vi "SEK2020v1VI1IrAteFinalDoCampo.vi"(8 "Parâmetros":T1={"Azul Max EV3 Cor"=17, "Azul Min EV3 Cor"=0, "Verde Max EV3 Cor"=6.0, "Verde Min EV3 Cor"=0.0, "Vermelho Max Ev3 Cor"=0, "Vermelho Min EV3 Cor"=0, "Chão EV3 Cor"=0.0, "Branco Max EV3 Cor"=0.0, "Branco Min EV3 Cor"=0.0, "Preto Max EV3 Cor"=0.0, "Preto Min EV3 Cor"=0.0, "Distância Tubulação"=0.0, "Distância Frontal"=0.0, "Amarelo Max EV3 Cor"=0.0, "Amarelo Min EV3 Cor"=0.0, "Distância Lateral"=0.0, "90°"=0.0, "180°"=0.0, "Seguidor de Linha"=0.0}, 10 "NXT/EV3":T2) -> (2 "NXT/EV3 2":T2)   [LabVIEW 2016]
uses:
  <vilib>/NXT/Subs/LVHSConnector.ctl
  <vilib>/NXT/LegoClasses/BrickReference/BrickReference.lvclass
  <vilib>/NXT/Block Support/NXT_OutputPort.ctl
  <vilib>/NXT/Block Support/NXT_InputPort.ctl
  <vilib>/NXT/Dual Mode Library/Sensors/EV3_Color_Reflect.vi
  <vilib>/NXT/NXTIO Xnodes/NXTIONodeSubVIs/NXTStopMotors.vi
  <vilib>/NXT/NXTIO Xnodes/AddressXNode/NXTIOAddress.xnode
  <vilib>/NXT/NXTIO Xnodes/NXTIOXNode/NXTIO.xnode
panel:
  # "Sensor EV3 Cor"
  # "Sensor Ultrassônico"
  # "Sensor Giroscópio"
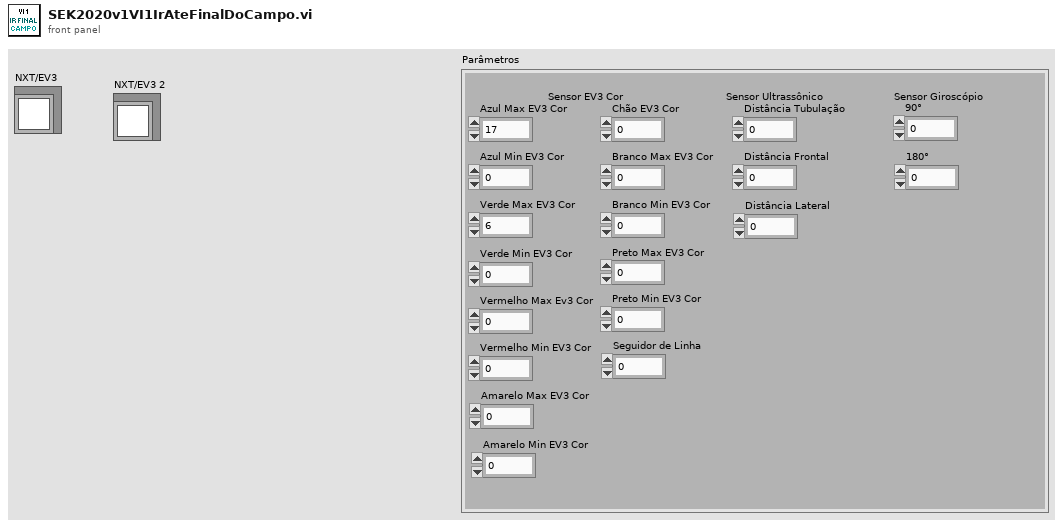
[diagram p1: front panel]
types:
  T1 = cluster{"Azul Max EV3 Cor":i32, "Azul Min EV3 Cor":i32, "Verde Max EV3 Cor":dbl, "Verde Min EV3 Cor":dbl, "Vermelho Max Ev3 Cor":i32, "Vermelho Min EV3 Cor":i32, "Chão EV3 Cor":sgl, "Branco Max EV3 Cor":sgl, "Branco Min EV3 Cor":sgl, "Preto Max EV3 Cor":sgl, "Preto Min EV3 Cor":sgl, "Distância Tubulação":sgl, "Distância Frontal":sgl, "Amarelo Max EV3 Cor":dbl, "Amarelo Min EV3 Cor":dbl, "Distância Lateral":sgl, "90°":sgl, "180°":sgl, "Seguidor de Linha":dbl}
  T2 = typedef "LVHSConnector.ctl" = refnum<class "BrickReference.lvclass">
  T3 = typedef "NXT_InputPort.ctl" = u32
  T4 = typedef "NXT_OutputPort.ctl" = u8
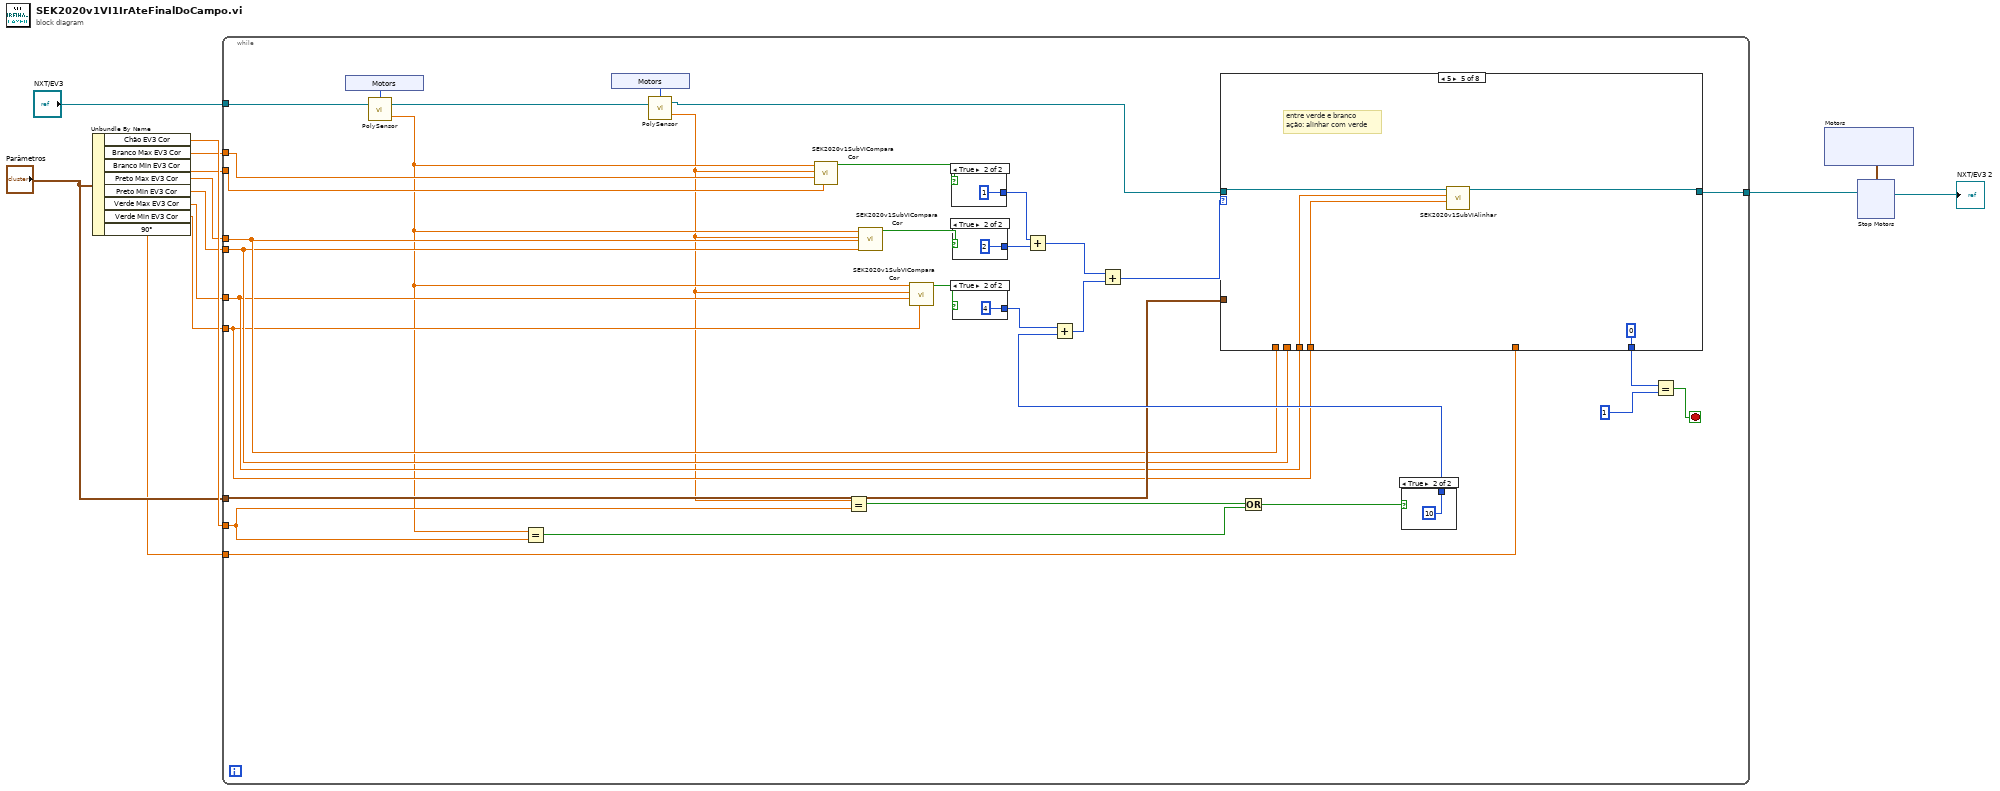
[diagram p0: block diagram]
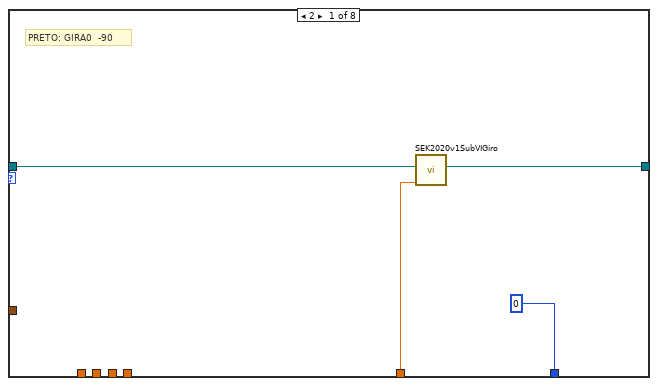
[diagram p2: hidden frame]
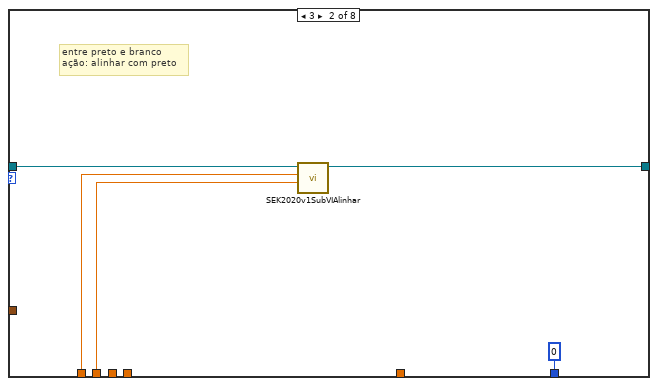
[diagram p3: hidden frame]
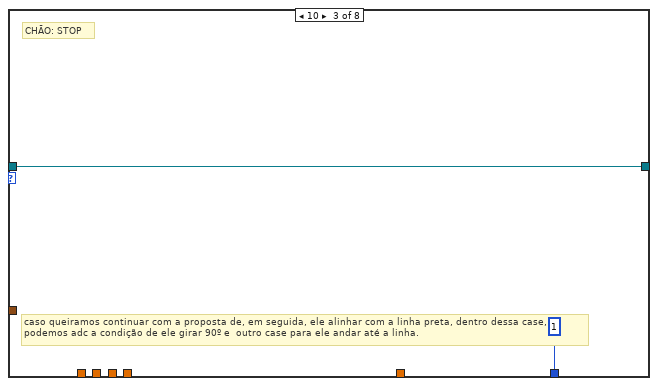
[diagram p4: hidden frame]
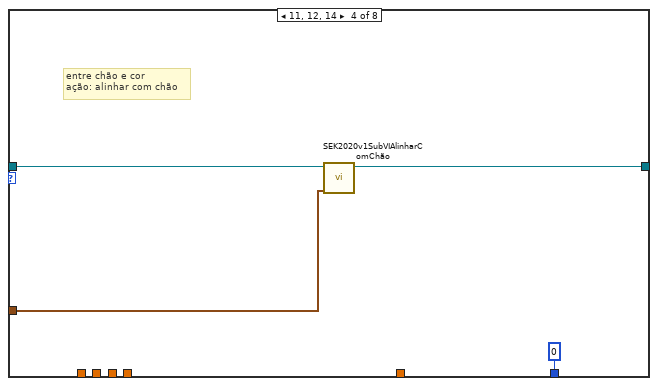
[diagram p5: hidden frame]
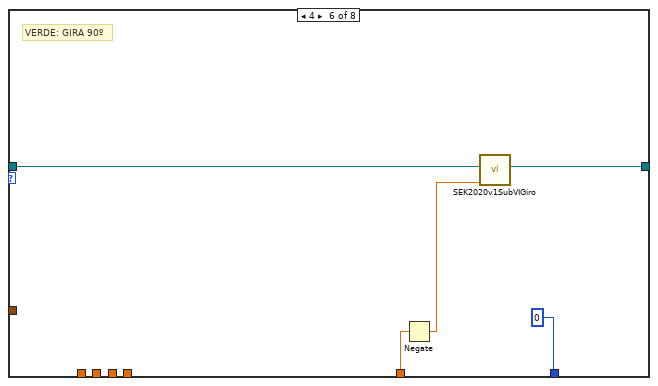
[diagram p6: hidden frame]
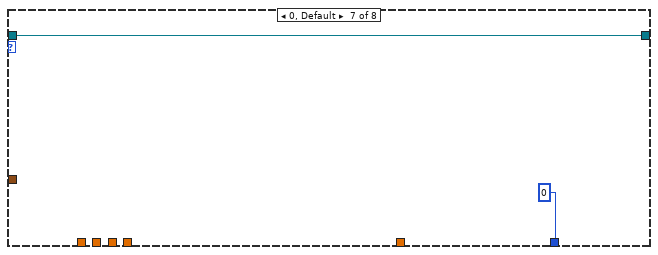
[diagram p7: hidden frame]
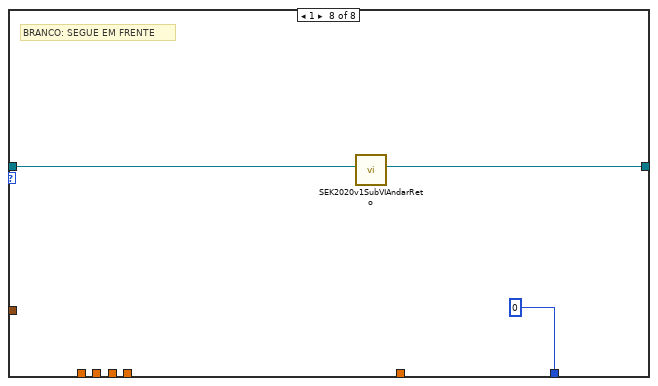
[diagram p8: hidden frame]
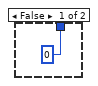
[diagram p9: hidden frame]
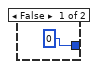
[diagram p10: hidden frame]
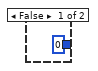
[diagram p11: hidden frame]
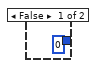
[diagram p12: hidden frame]
diagram:
  n1 = Unbundle By Name("Parâmetros") -> ("Chão EV3 Cor"=w12:sgl, "Branco Max EV3 Cor"=w5:sgl, "Branco Min EV3 Cor"=w8:sgl, "Preto Max EV3 Cor"=w4:sgl, "Preto Min EV3 Cor"=w7:sgl, "Verde Max EV3 Cor"=w3:dbl, "Verde Min EV3 Cor"=w6:dbl, "90°"=w1:sgl)
  n2 = while {
    tunnel: "NXT/EV3" -> [w34]
    tunnel: w12 -> [w21]
    tunnel: [w37] -> w9
    tunnel: w8 -> [w24]
    tunnel: w7 -> [w22]
    tunnel: w6 -> [w18]
    tunnel: w5 -> [w25]
    tunnel: w4 -> [w23]
    tunnel: w3 -> [w19]
    tunnel: "Parâmetros" -> [w26]
    tunnel: w1 -> [w14]
    stop <- w33 stop-if-true
    n3 = xnode "Motors"() -> ("Sensor"=w45:T3)
    n4 = call-poly <vilib>:"PolySensor.vi"("NXT/EV3"=w34, "Port (Port 1)"=w45) -> ("Scaled Value"=w17:sgl, "NXT/EV3"=w35:T2)  [unwired: 1 in]
    n5 = Equal?(x=w17, y=w21) -> (x = y?=w32:bool)
    n6 = xnode "Motors"() -> ("Sensor"=w46:T3)
    n7 = call-poly <vilib>:"PolySensor.vi"("NXT/EV3"=w35, "Port (Port 1)"=w46) -> ("Scaled Value"=w16:sgl, "NXT/EV3"=w15:T2)  [unwired: 1 in]
    n8 = call "SEK2020v1SubVIComparaCor.vi"("Branco Min EV3 Cor"=w24, "Branco Max EV3 Cor"=w25, "Scaled Value 2"=w16, "Scaled Value"=w17) -> ("Boolean"=w29:bool)  [unwired: 7 in]
    n9 = Equal?(x=w16, y=w21) -> (x = y?=w44:bool)
    n10 = call "SEK2020v1SubVIComparaCor.vi"("Branco Min EV3 Cor"=w22, "Branco Max EV3 Cor"=w23, "Scaled Value 2"=w16, "Scaled Value"=w17) -> ("Boolean"=w28:bool)  [unwired: 7 in]
    n11 = call "SEK2020v1SubVIComparaCor.vi"("Branco Min EV3 Cor"=w18, "Branco Max EV3 Cor"=w19, "Scaled Value 2"=w16, "Scaled Value"=w17) -> ("Boolean"=w27:bool)  [unwired: 7 in]
    n12 = case shown="True" w29 {
      tunnel: [0 1] -> w43
      frame False {
      }
      frame True {
      }
    }
    n13 = case shown="True" w28 {
      tunnel: [0 2] -> w42
      frame False {
      }
      frame True {
      }
    }
    n14 = case shown="True" w27 {
      tunnel: [0 4] -> w38
      frame False {
      }
      frame True {
      }
    }
    n15 = Add(x=w43, y=w42) -> (x+y=w39:i32)
    n16 = Or(x=w44, y=w32) -> (x .or. y?=w36:bool)
    n17 = case shown="True" w36 {
      tunnel: [0 10] -> w41
      frame False {
      }
      frame True {
      }
    }
    n18 = Add(x=w38, y=w41) -> (x+y=w40:i32)
    n19 = Add(x=w39, y=w40) -> (x+y=w20:i32)
    n20 = case shown="5" w20 {
      tunnel: [w49 w53 w56 w61 w66 w70 w72 w75] -> w37
      tunnel: [0 0 1 0 0 0 0 0] -> w30
      tunnel: w23 -> [_ w55 _ _ _ _ _ _]
      tunnel: w22 -> [_ w54 _ _ _ _ _ _]
      tunnel: w26 -> [_ _ _ w60 _ _ _ _]
      tunnel: w19 -> [_ _ _ _ w65 _ _ _]
      tunnel: w18 -> [_ _ _ _ w64 _ _ _]
      tunnel: w15 -> [w48 w51 w56 w58 w62 w69 w72 w74]
      tunnel: w14 -> [w47 _ _ _ _ w68 _ _]
      frame 2 {
        # "PRETO: GIRA0  -90"
        n21 = call "SEK2020v1SubVIGiro.vi"("ANGULO"=w47, "NXT/EV3"=w48) -> ("NXT/EV3 2"=w49:T2)  [unwired: 7 in]
      }
      frame 3 {
        # "entre preto e branco\nação: alinhar com preto"
        n22 = call "SEK2020v1SubVIAlinhar.vi"("Min EV3 Cor"=w54, "Max EV3 Cor"=w55, "NXT/EV3"=w51) -> ("NXT/EV3 2"=w53:T2)  [unwired: 8 in]
      }
      frame 10 {
        # "caso queiramos continuar com a proposta de, em seguida, ele alinhar com a linha preta, dentro dessa case,\npodemos adc a condição de ele girar 90º e  outro case para ele andar até a linha."
        # "CHÃO: STOP"
      }
      frame 11, 12, 14 {
        # "entre chão e cor\nação: alinhar com chão"
        n23 = call "SEK2020v1SubVIAlinharComChão.vi"("Parâmetros"=w60, "NXT/EV3"=w58) -> ("NXT/EV3 2"=w61:T2)  [unwired: 9 in]
      }
      frame 5 {
        # "entre verde e branco\nação: alinhar com verde"
        n24 = call "SEK2020v1SubVIAlinhar.vi"("Min EV3 Cor"=w64, "Max EV3 Cor"=w65, "NXT/EV3"=w62) -> ("NXT/EV3 2"=w66:T2)  [unwired: 8 in]
      }
      frame 4 {
        # "VERDE: GIRA 90º"
        n25 = Negate(x=w68) -> (-x=w67:sgl)
        n26 = call "SEK2020v1SubVIGiro.vi"("ANGULO"=w67, "NXT/EV3"=w69) -> ("NXT/EV3 2"=w70:T2)  [unwired: 7 in]
      }
      frame 0, Default {
      }
      frame 1 {
        # "BRANCO: SEGUE EM FRENTE"
        n27 = call "SEK2020v1SubVIAndarReto.vi"("NXT/EV3"=w74) -> ("NXT/EV3 2"=w75:T2)  [unwired: 9 in]
      }
    }
    n28 = Equal?(x=w30, y=1) -> (x = y?=w33:bool)
  }
  n29 = xnode "Motors"() -> ("Motor"=w11:cluster{"Port":T4, "Port":T4})
  n30 = xnode "Stop Motors"("Motors"=w11, "NXT/EV3"=w9) -> ("NXT/EV3"=→"NXT/EV3 2":T2)
